vi "I2C Get Channel Info.vi"(0 "index":u32, 11 "error in (no error)":errorcluster) -> (3 "Flags":u32, 4 "ftHandle":u32, 6 "LocId":u32, 8 "ID":u32, 10 "Type":u32, 13 "Description":string, 14 "Serial number":string, 15 "error out":errorcluster)   [LabVIEW 2017, in "libMPSSE.lvlib"]
doc: "FTDI_API FT_STATUS I2C_GetChannelInfo(uint32 index, \n FT_DEVICE_LIST_INFO_NODE *chanInfo);"
uses:
  libMPSSE.lvlib
  \\Mac\Home/Desktop/libMPSSE-SPI-LabVIEW-master/libMPSSE.dll
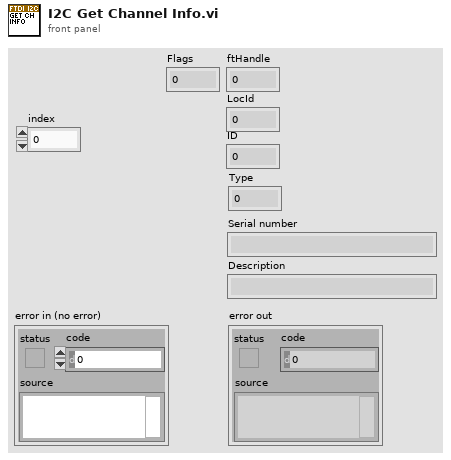
[diagram p1: front panel]
types:
  T1 = cluster{"Flags":u32, "Type":u32, "ID":u32, "LocId":u32, "SerialNumber[0]":i8, "SerialNumber[1]":i8, "SerialNumber[2]":i8, "SerialNumber[3]":i8, "SerialNumber[4]":i8, "SerialNumber[5]":i8, "SerialNumber[6]":i8, "SerialNumber[7]":i8, "SerialNumber[8]":i8, "SerialNumber[9]":i8, "SerialNumber[10]":i8, "SerialNumber[11]":i8, "SerialNumber[12]":i8, "SerialNumber[13]":i8, "SerialNumber[14]":i8, "SerialNumber[15]":i8, "Description[0]":i8, "Description[1]":i8, "Description[2]":i8, "Description[3]":i8, "Description[4]":i8, "Description[5]":i8, "Description[6]":i8, "Description[7]":i8, "Description[8]":i8, "Description[9]":i8, "Description[10]":i8, "Description[11]":i8, "Description[12]":i8, "Description[13]":i8, "Description[14]":i8, "Description[15]":i8, "Description[16]":i8, "Description[17]":i8, "Description[18]":i8, "Description[19]":i8, "Description[20]":i8, "Description[21]":i8, "Description[22]":i8, "Description[23]":i8, "Description[24]":i8, "Description[25]":i8, "Description[26]":i8, "Description[27]":i8, "Description[28]":i8, "Description[29]":i8, "Description[30]":i8, "Description[31]":i8, "Description[32]":i8, "Description[33]":i8, "Description[34]":i8, "Description[35]":i8, "Description[36]":i8, "Description[37]":i8, "Description[38]":i8, "Description[39]":i8, "Description[40]":i8, "Description[41]":i8, "Description[42]":i8, "Description[43]":i8, "Description[44]":i8, "Description[45]":i8, "Description[46]":i8, "Description[47]":i8, "Description[48]":i8, "Description[49]":i8, "Description[50]":i8, "Description[51]":i8, "Description[52]":i8, "Description[53]":i8, "Description[54]":i8, "Description[55]":i8, "Description[56]":i8, "Description[57]":i8, "Description[58]":i8, "Description[59]":i8, "Description[60]":i8, "Description[61]":i8, "Description[62]":i8, "Description[63]":i8, "ftHandle":u32}
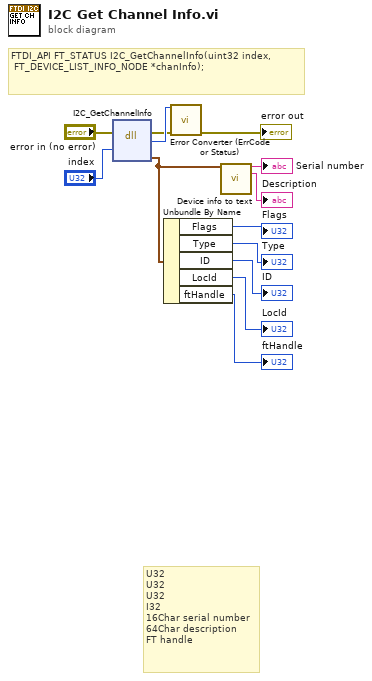
[diagram p0: block diagram]
diagram:
  # "U32\nU32\nU32\nI32\n16Char serial number\n64Char description\nFT handle"
  # "FTDI_API FT_STATUS I2C_GetChannelInfo(uint32 index, \n\tFT_DEVICE_LIST_INFO_NODE *chanInfo);"
  n1 = dll-call lib="\\\\Mac\\Home/Desktop/libMPSSE-SPI-LabVIEW-master/libMPSSE.dll" fn="I2C_GetChannelInfo"(error in="error in (no error)", "index"="index") -> (error out=w10:errorcluster, "return type"=w13:u32, "chanInfo out"=w6:T1)  [unwired: 4 in, 1 out]
  n2 = Unbundle By Name(w6) -> ("Flags"=→"Flags":u32, "Type"=→"Type":u32, "ID"=→"ID":u32, "LocId"=→"LocId":u32, "ftHandle"=→"ftHandle":u32)
  n3 = call "Error Converter (ErrCode or Status).vi"("error code"=w13, "error in (no error)"=w10) -> ("error out"=→"error out":errorcluster)  [unwired: 13 in]
  n4 = call "Device info to text.vi"("chanInfo out"=w6) -> ("Serial number"=→"Serial number":string, "Description"=→"Description":string)  [unwired: 13 in]
